vi "Arm Hardware.vi"(8 "error in (no error)":errorcluster, 9 "Request type":T1=enum."User command", 11 "RP I-V Driver in":refnum<class "RP I-V Driver.lvclass">) -> (0 "error out":errorcluster, 3 "RP I-V Driver out":refnum<class "RP I-V Driver.lvclass">)   [LabVIEW 2024, in "RP I-V Driver.lvclass"]
uses:
  RP I-V Driver.lvclass
  LabActor/Controllers/Process Controller/Request type.ctl
  RP Command.ctl
  Red Pitaya Digitizer/Red Pitaya Digitizer.lvclass/Red Pitaya Digitizer.ctl
  RP I-V Driver.lvclass/RP I-V Driver.ctl
  Red Pitaya Digitizer/Read Logic tag.vi
  Write Output waveform.vi
  RP Instrument/RP Instrument.lvclass
  Red Pitaya Digitizer/Red Pitaya Digitizer.lvclass
panel:
  out "Status response 2":u32=1 format="0x%x (%d)"
  out "Status response":u32=1 format="0x%x (%d)"
  out "Finished 2":bool
  out "Armed 2":bool
  out "Finished":bool
  out "Armed":bool
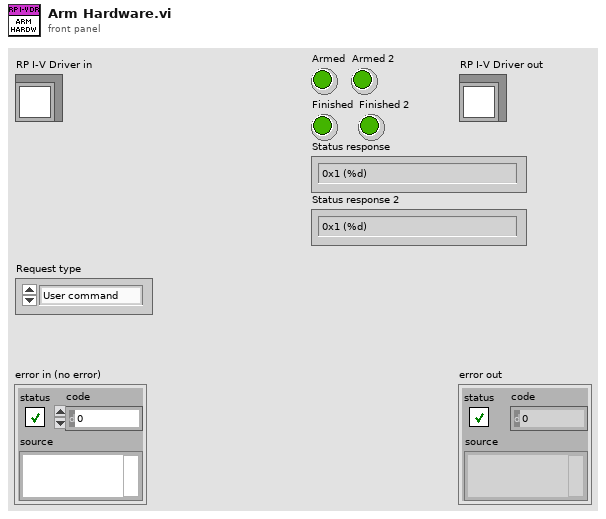
[diagram p1: front panel]
types:
  T1 = typedef "Request type.ctl" = enum16{"Process complete", "User command", "Auto-restart", "Error"}
  T2 = typedef "RP Command.ctl" = enum16{"Reset", "Read IDN", "Stop server", "Get status", "Get temperature", "Connect client", "Arm", "Software trigger", "Get whole buffer", "Get chunk", "System call", "Get config", "Set config", "Recieve data", "Recieve Calibartion", "Transmit data"}
  T3 = typedef "RP I-V Configuration.ctl" = cluster{"I-V parameters":T4, "Ranges":dbl[], "Post-trigger delay":dbl, "Post-trigger duration":dbl, "Output delay":dbl}
  T4 = typedef "I-V parameters.ctl" = cluster{"Start magnitude":dbl, "Magnitude increment":dbl, "End magnitude":dbl, "Ramp length":i32, "Top  length":i32, "Threshold ":dbl, "Processing delay":u16, "Output gain ":dbl, "Interpolation":i32, "Stop after":u16, "Detector window":i32}
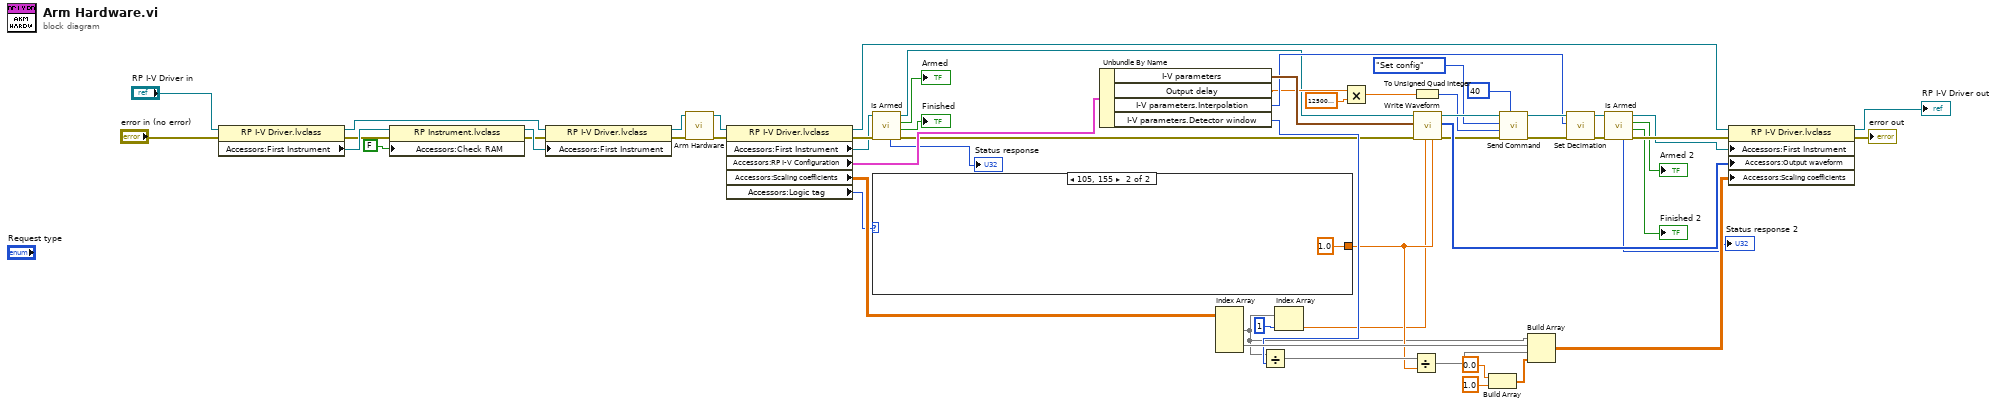
[diagram p0: block diagram]
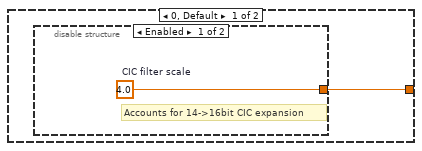
[diagram p2: hidden frame]
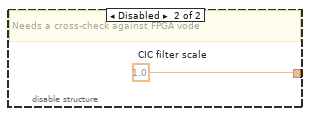
[diagram p3: hidden frame]
diagram:
  n1 = property class="RP I-V Driver.lvclass"(reference="RP I-V Driver in", error in="error in (no error)") -> (reference out=w8:refnum<class "RP I-V Driver.lvclass">, error out=w5:errorcluster, "Accessors:First Instrument"=w9:refnum<class "RP Instrument.lvclass">)
  n2 = property class="RP Instrument.lvclass"(reference=w9, error in=w5, "Accessors:Check RAM"=FALSE ("Check RAM")) -> (reference out=w10:refnum<class "RP Instrument.lvclass">, error out=w6:errorcluster)
  n3 = property class="RP I-V Driver.lvclass"(reference=w8, error in=w6, "Accessors:First Instrument"=w10) -> (reference out=w7:refnum<class "RP I-V Driver.lvclass">, error out=w3:errorcluster)
  n4 = call-parent "Arm Hardware.vi"("error in (no error)"=w3, "Red Pitaya Digitizer in"=w7) -> ("error out"=w46:errorcluster, "Red Pitaya Digitizer out"=w45:refnum<class "RP I-V Driver.lvclass">)  [unwired: 8 in]
  n5 = property class="RP I-V Driver.lvclass"(reference=w45, error in=w46) -> (reference out=w57:refnum<class "RP I-V Driver.lvclass">, error out=w30:errorcluster, "Accessors:First Instrument"=w12:refnum<class "RP Instrument.lvclass">, "Accessors:RP I-V Configuration"=w51:T3, "Accessors:Scaling coefficients"=w39:dbl[][], "Accessors:Logic tag"=w17:u16)
  n6 = call-dynamic "Is Armed.vi"("error in (no error)"=w30, "RP Instrument in"=w12) -> ("error out"=w29:errorcluster, "Finished"=→"Finished":bool, "Armed"=→"Armed":bool, "RP Instrument out"=w28:refnum<class "RP Instrument.lvclass">, "Status response"=→"Status response":u32)  [unwired: 5 in]
  n7 = case shown="105, 155" w17 {
    tunnel: [w58 1.0 ("CIC filter scale")] -> w15
    frame 0, Default {
      n8 = disable-structure shown="Enabled" {
        disable-tunnel: [w59 w60] -> w58
        frame Enabled {
          w59 = 4.0  # CIC filter scale
          # "Accounts for 14->16bit CIC expansion"
        }
        frame Disabled {
          w60 = 1.0  # CIC filter scale
          # "Needs a cross-check against FPGA vode"
        }
      }
    }
    frame 105, 155 {
    }
  }
  n9 = Unbundle By Name(w51) -> ("I-V parameters"=w50:T4, "Output delay"=w32:dbl, "I-V parameters.Interpolation"=w40:i32, "I-V parameters.Detector window"=w37:i32)
  n10 = Index Array(array=w39) -> (element #1=w13:dbl[], element #2=w38:dbl[])  [unwired: 4 in]
  n11 = Divide(x=w13, y=w37) -> (x/y=w31:dbl[])
  n12 = Index Array(array=w13, index=1) -> (element=w14:dbl)
  n13 = Multiply(x=w32, y=125000000.0) -> (x*y=w48:dbl)
  n14 = Divide(x=w31, y=w15) -> (x/y=w1:dbl[])
  n15 = To Unsigned Quad Integer(1:w48) -> (0:w47:u64)
  n16 = call-dynamic "Write Waveform.vi"("CIC filter factor"=w15, "Input scale"=w14, "error in (no error)"=w29, "I-V parameters"=w50, "RP Instrument in"=w28) -> ("error out"=w54:errorcluster, "Output Waveform"=w56:i16[], "RP Instrument out"=w55:refnum<class "RP Instrument.lvclass">)  [unwired: 4 in]
  n17 = Build Array(0.0 ("element"), 1.0 ("element")) -> (w34:dbl[])
  n18 = call-dynamic "Send Command.vi"("Config offset"=u64 40, "error in (no error)"=w54, "Command payload"=w47, "Command number"=RP_Command."Set config", "RP Instrument in"=w55) -> ("error out"=w41:errorcluster, "RP Instrument out"=w42:refnum<class "RP Instrument.lvclass">)  [unwired: 5 in]
  n19 = Build Array(w13, w38, w1, w34) -> (w33:dbl[][])
  n20 = call-dynamic "Set Decimation.vi"("error in (no error)"=w41, "Decimation"=w40, "RP Instrument in"=w42) -> ("error out"=w24:errorcluster, "RP Instrument out"=w23:refnum<class "RP Instrument.lvclass">)  [unwired: 7 in]
  n21 = call-dynamic "Is Armed.vi"("error in (no error)"=w24, "RP Instrument in"=w23) -> ("error out"=w25:errorcluster, "Finished"=→"Finished 2":bool, "Armed"=→"Armed 2":bool, "RP Instrument out"=w22:refnum<class "RP Instrument.lvclass">, "Status response"=→"Status response 2":u32)  [unwired: 5 in]
  n22 = property class="RP I-V Driver.lvclass"(reference=w57, error in=w25, "Accessors:First Instrument"=w22, "Accessors:Output waveform"=w56, "Accessors:Scaling coefficients"=w33) -> (reference out=→"RP I-V Driver out":refnum<class "RP I-V Driver.lvclass">, error out=→"error out":errorcluster)
